vi "2_TDMS.vi"() -> ()   [LabVIEW 2014]
panel:
  out "Group 2 channels":string[](array[string])=["Random 1", "Random 2"]
  out "Group 1 channels":string[](array[string])=["Random 1", "Random 2"]
  out "TDMS data read":dbl[][](graph)
  out "property names":string[](array[string])
  out "property values":variant[](array[variant])
  out "Channels read":string[](array[string])
  in  "Group to read":string="Random"
  in  "Group 2":string="Others"
  in  "Group 1":string="Random"
  in  "Title":string="My measurements"
  in  "Generate":bool
  in  "stop":bool
  in  "Load":bool
  in  "Save":bool
  out "Generated data":dbl[][](graph)
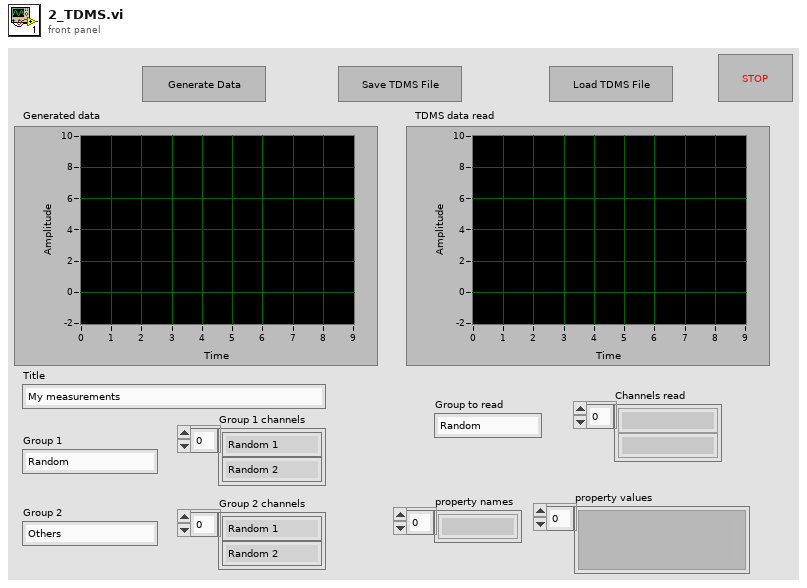
[diagram p1: front panel]
types:
  T1 = enum16{"open", "open or create", "create or replace", "create", "open (read-only)"}
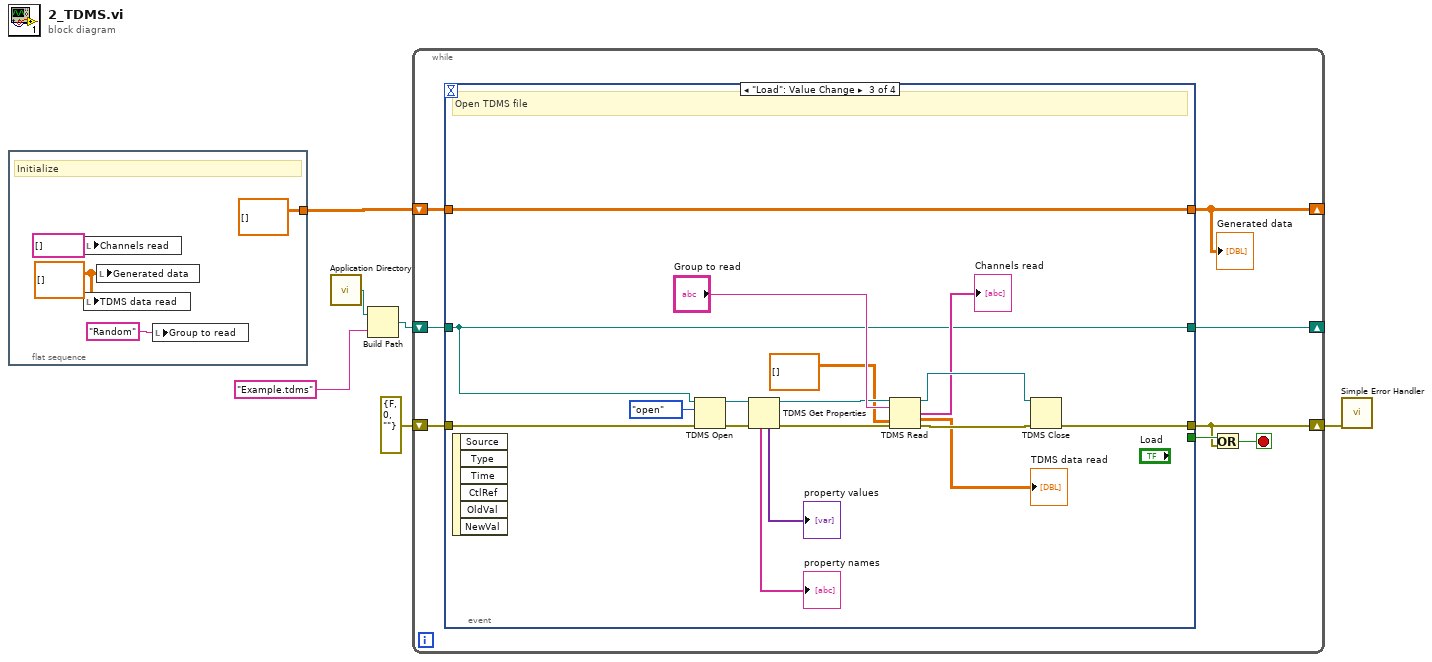
[diagram p0: block diagram]
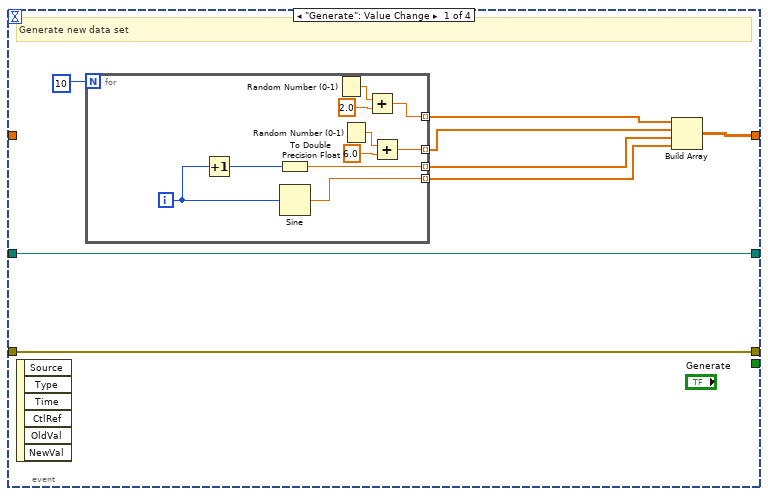
[diagram p2: hidden frame]
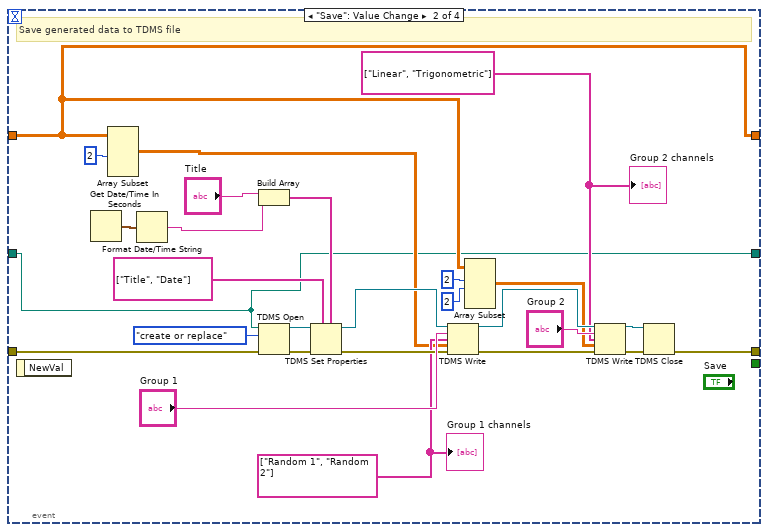
[diagram p3: hidden frame]
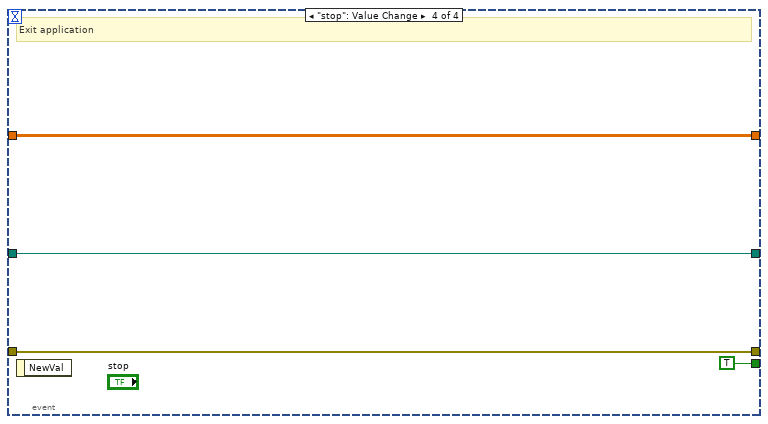
[diagram p4: hidden frame]
diagram:
  n1 = flat-sequence {
    tunnel: [dbl[][] []] -> w4
    frame #0 {
      w7 = dbl[][] [] ("Generated data")
      # "Initialize"
      n2 = local write "Channels read"(string[] [] ("Channels")) -> ()
      n3 = local write "TDMS data read"(w7) -> ()
      n4 = local write "Generated data"(w7) -> ()
      n5 = local write "Group to read"("Random" ("group name in")) -> ()
    }
  }
  n6 = call <vilib>:"Application Directory.vi"() -> ("Application Directory"=w2:path)
  n7 = Build Path(base path=w2, name or relative path="Example.tdms") -> (appended path=w3:path)
  n8 = while {
    shift-right: [w17] -> _
    shift-left: w4 -> [w18]
    shift-right: [w14] -> w5
    shift-left: errorcluster {"status"=FALSE, "code"=0, "source"=""} ("error constant") -> [w16]
    shift-right: [w12] -> _
    shift-left: w3 -> [w11]
    stop <- w13 stop-if-true
    n9 = event shown="[2] \"Load\": Value Change" {
      selector: _ -> [_ _ _ _]
      dyn-events: _ -> [_ _ _ _]
      timeout: _ -> [_ _ _ _]
      tunnel: [_ _ _ TRUE] -> w15
      tunnel: [w20 w40 w75 w82] -> w17
      tunnel: w18 -> [_ w40 w75 w82]
      tunnel: w16 -> [w23 w56 w77 w83]
      tunnel: [w23 w55 w76 w83] -> w14
      tunnel: [w19 w37 w64 w81] -> w12
      tunnel: w11 -> [w19 w37 w64 w81]
      event "Generate": Value Change {
        # "Generate new data set"
        n10 = event-data() -> ()  [unwired: 1 in, 6 out]
        n11 = for {
          N: 10 -> [_]
          tunnel: [w31] -> w25 mode=indexing
          tunnel: [w35] -> w26 mode=indexing
          tunnel: [w34] -> w22 mode=indexing
          tunnel: [w27] -> w21 mode=indexing
          i -> [w30]
          n12 = Increment(x=w30) -> (x+1=w36:i32)
          n13 = To Double Precision Float(number=w36) -> (double precision float=w35:dbl)
          n14 = Sine(x=w30) -> (sin(x)=w34:dbl)
          n15 = Random Number (0-1)() -> (number: 0 to 1=w28:dbl)
          n16 = Random Number (0-1)() -> (number: 0 to 1=w33:dbl)
          n17 = Add(x=w28, y=2.0) -> (x+y=w27:dbl)
          n18 = Add(x=w33, y=6.0) -> (x+y=w31:dbl)
        }
        n19 = Build Array(w21, w25, w26, w22) -> (w20:dbl[][])
      }
      event "Save": Value Change {
        w38 = string[] ["Linear", "Trigonometric"] ("property names")
        w45 = string[] ["Random 1", "Random 2"] ("property names")
        # "Save generated data to TDMS file"
        n20 = event-data() -> ()  [unwired: 1 in, 1 out]
        n21 = Get Date/Time In Seconds() -> (seconds since 1Jan1904=w54:timestamp)
        n22 = Array Subset(array=w40, length (row)=2 ("length")) -> (w44:dbl[][])  [unwired: 3 in]
        n23 = Format Date/Time String(seconds (now)=w54) -> (date/time string=w52:string)  [unwired: 2 in]
        n24 = Build Array("Title", w52) -> (w51:string[])
        n25 = TDMS Open(8:w56, 10:T1."create or replace" ("operation (0:open)"), 11:w37) -> (0:w57:errorcluster, 3:w60:refnum<k34>)  [unwired: 4 in]
        n26 = TDMS Set Properties(5:w51, 7:string[] ["Title", "Date"] ("property names"), 8:w57, 11:w60) -> (0:w58:errorcluster, 3:w59:refnum<k34>)  [unwired: 2 in, 2 out]
        n27 = TDMS Write(0:w59, 5:"Group 1", 7:w45, 9:w44, 11:w58) -> (4:w50:refnum<k34>, 15:w49:errorcluster)  [unwired: 1 in, 2 out]
        n28 = Array Subset(array=w40, index (row)=2 ("index"), length (row)=2 ("length")) -> (w43:dbl[][])  [unwired: 2 in]
        n29 = TDMS Write(0:w50, 5:"Group 2", 7:w38, 9:w43, 11:w49) -> (4:w48:refnum<k34>, 15:w47:errorcluster)  [unwired: 1 in, 2 out]
        n30 = TDMS Close(8:w47, 11:w48) -> (0:w55:errorcluster)  [unwired: 1 out]
        "Group 1 channels" <- w45
        "Group 2 channels" <- w38
      }
      event "Load": Value Change {
        # "Open TDMS file"
        n31 = event-data() -> ()  [unwired: 1 in, 6 out]
        n32 = TDMS Open(8:w77, 10:T1."open" ("operation (0:open)"), 11:w64) -> (0:w71:errorcluster, 3:w72:refnum<k34>)  [unwired: 4 in]
        n33 = TDMS Get Properties(8:w71, 11:w72) -> (0:w69:errorcluster, 3:w70:refnum<k34>, 4:→"property values":variant[], 6:→"property names":string[])  [unwired: 4 in, 2 out]
        n34 = TDMS Read(0:w70, 5:"Group to read", 11:w69, 12:dbl[][] []) -> (4:w79:refnum<k34>, 8:→"Channels read":string[], 10:→"TDMS data read":dbl[][], 15:w78:errorcluster)  [unwired: 4 in, 2 out]
        n35 = TDMS Close(8:w78, 11:w79) -> (0:w76:errorcluster)  [unwired: 1 out]
      }
      event "stop": Value Change {
        # "Exit application"
        n36 = event-data() -> ()  [unwired: 1 in, 1 out]
      }
    }
    "Generated data" <- w17
    n37 = Or(x=w15, y=w14) -> (x .or. y?=w13:bool)
  }
  n38 = call <vilib>:"Simple Error Handler.vi"("error in (no error)"=w5) -> ()  [unwired: 4 in, 5 out]
